vi "Stop Logic-Imaging.vi"(8 "error in (no error)":errorcluster, 11 "UI queue":refnum<queue>) -> (0 "error out":errorcluster)   [LabVIEW 2013]
uses:
  Queue/Message Queue/Typedefs/Message Cluster.ctl
  Typedefs/Read Write Enum.ctl
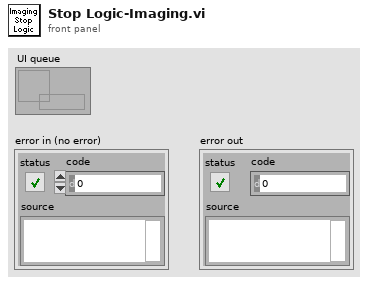
[diagram p1: front panel]
types:
  T1 = typedef "Read Write Enum.ctl" = enum16{"Read", "Write"}
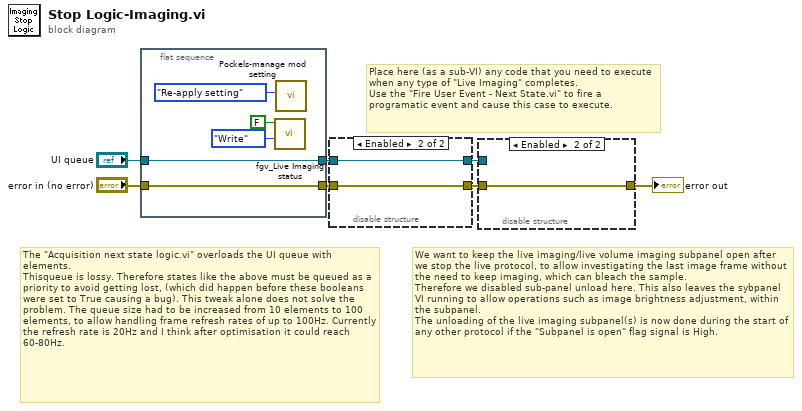
[diagram p0: block diagram]
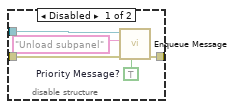
[diagram p2: hidden frame]
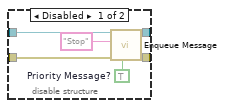
[diagram p3: hidden frame]
diagram:
  # "We want to keep the live imaging/live volume imaging subpanel open after we stop the live protocol, to allow investigating the last image frame without the need to keep imaging, which can bleach the sample.\nTherefore we disabled sub-panel unload here. This also leaves the sybpanel VI running to allow operations such as image brightness adjustment, within the subpanel.\nThe unloading of the live imaging subpanel(s) is now done during the start of any other protocol if the \"Subpanel is open\" flag signal is High."
  # "The \"Acquisition next state logic.vi\" overloads the UI queue with elements.\nThisqueue is lossy. Therefore states like the above must be queued as a priority to avoid getting lost, (which did happen before these booleans were set to True causing a bug). This tweak alone does not solve the problem. The queue size had to be increased from 10 elements to 100 elements, to allow handling frame refresh rates of up to 100Hz. Currently the refresh rate is 20Hz and I think after optimisation it could reach 60-80Hz."
  # "Place here (as a sub-VI) any code that you need to execute when any type of \"Live Imaging\" completes.\nUse the \"Fire User Event - Next State.vi\" to fire a programatic event and cause this case to execute."
  n1 = flat-sequence {
    tunnel: "UI queue" -> [w12]
    tunnel: [w12] -> w4
    tunnel: [w11] -> w2
    tunnel: "error in (no error)" -> [w11]
    frame #0 {
      n2 = call "fgv_Live Imaging status.vi"("Function"=Read_Write_Enum."Write", "Live Imaging?"=FALSE ("Timelapse?")) -> ()  [unwired: 8 in, 2 out]
      n3 = call "Pockels-manage mod setting.vi"("Function"=enum16{"Capture setting", "Re-apply setting"}."Re-apply setting") -> ()  [unwired: 10 in, 1 out]
    }
  }
  n4 = disable-structure shown="Enabled" {
    disable-tunnel: [w18 w20] -> w7
    disable-tunnel: [w17 w19] -> w6
    disable-tunnel: w4 -> [w14 w20]
    disable-tunnel: w2 -> [w13 w19]
    frame Disabled {
      w15 = TRUE  # Priority Message?
      n5 = call "Enqueue Message.vi"("Priority Message? (F)"=w15, "error in (no error)"=w13, "Message"="Stop", "Queue"=w14) -> ("error out"=w17:errorcluster, "Queue out"=w18:refnum<queue>)  [unwired: 6 in]
    }
    frame Enabled {
    }
  }
  n6 = disable-structure shown="Enabled" {
    disable-tunnel: w7 -> [w25 _]
    disable-tunnel: w6 -> [w24 w26]
    disable-tunnel: [w23 w26] -> w1
    frame Disabled {
      w21 = TRUE  # Priority Message?
      n7 = call "Enqueue Message.vi"("Priority Message? (F)"=w21, "error in (no error)"=w24, "Message"="Unload subpanel", "Queue"=w25) -> ("error out"=w23:errorcluster)  [unwired: 6 in, 1 out]
    }
    frame Enabled {
    }
  }
  "error out" <- w1
